vi "Configure Byte Order.vi"(0 "VISA resource name":refnum<visa-resource-name>, 5 "Byte Order":u16(ring) items=["Normal", "Swapped"], 11 "error in (no error)":errorcluster) -> (4 "VISA resource name out":refnum<visa-resource-name>, 15 "error out":errorcluster)   [LabVIEW 2020, in "Keithley DMM6500 DAQ6500 Series.lvlib"]
doc: "Sets the byte order for the IEEE-754 binary formats. Swapped is equivalent to little-endian; Normal is equivalent to big-endian."
uses:
  <instrlib>/Keithley DMM6500 DAQ6500 Series/Keithley DMM6500 DAQ6500 Series.lvlib
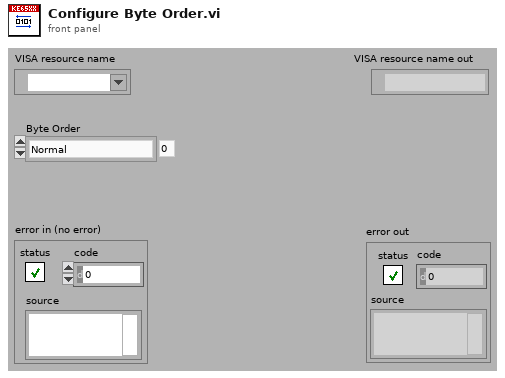
[diagram p1: front panel]
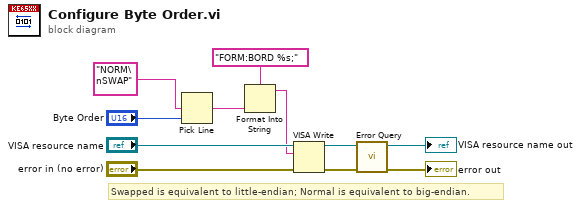
[diagram p0: block diagram]
diagram:
  # "Swapped is equivalent to little-endian; Normal is equivalent to big-endian."
  n1 = Pick Line(multi-line string="NORM\nSWAP", line index="Byte Order") -> (output string=w3:string)  [unwired: 1 in]
  n2 = Format Into String(format string="FORM:BORD %s;", w3) -> (resulting string=w5:string)  [unwired: 2 in, 1 out]
  n3 = VISA Write(VISA resource name="VISA resource name", write buffer=w5, error in (no error)="error in (no error)") -> (VISA resource name out=w9:refnum<visa-resource-name>, error out=w8:errorcluster)  [unwired: 1 out]
  n4 = call <instrlib>:"Error Query.vi"("error in (no error)"=w8, "VISA resource name"=w9) -> ("error out"=→"error out":errorcluster, "VISA resource name out"=→"VISA resource name out":refnum<visa-resource-name>)  [unwired: 6 in, 2 out]
